vi "[FGV]PEMG.vi"(1 "Select":enum16{"READ", "WRITE"}(ring), 2 "Array":dbl[](array[numeric])) -> (0 "Array 2":dbl[](array[numeric]))   [LabVIEW 2018]
panel:
  out "error out":errorcluster
  in  "error in":errorcluster
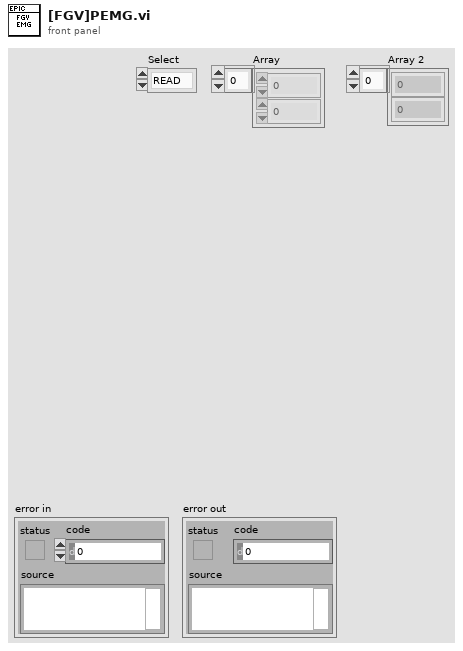
[diagram p1: front panel]
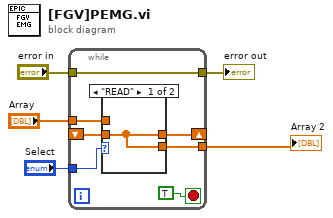
[diagram p0: block diagram]
diagram:
  n1 = while {
    tunnel: "Select" -> [w12]
    tunnel: [w11] -> w3
    tunnel: "error in" -> [w11]
    tunnel: [w10] -> w1
    shift-right: [w9] -> _
    shift-left: _ -> [w8]
    tunnel: "Array" -> [w7]
    stop <- TRUE stop-if-true
    n2 = case shown="\"READ\"" w12 {
      tunnel: w8 -> [w13 _]
      tunnel: [w13 w14] -> w10
      tunnel: [w13 w14] -> w9
      tunnel: w7 -> [_ w14]
      frame "READ" {
      }
      frame "WRITE" {
      }
    }
  }
  "error out" <- w3
  "Array 2" <- w1
